vi "Periodic Tasks.vi"(8 "error in":errorcluster) -> ()   [LabVIEW 2017]
doc: "This VI runs in parallel to other robot code. It can contain as many user-defined periodic loops as you need. These can carry out PID or other sorts of timed response."
uses:
  d7755982-491b-4a48-a7ae-66e749655537.vi
  <vilib>/Rock Robotics/WPI/Utilities/WPI_GetSetVariantRefNum.vi
  <vilib>/Rock Robotics/Network Tables/NT Write Boolean.vi
  <vilib>/Rock Robotics/Network Tables/NT Write Number.vi
  <vilib>/Rock Robotics/Network Tables/NT Write Numeric Array.vi
  <vilib>/Rock Robotics/Network Tables/NT Write Boolean Array.vi
  <vilib>/Rock Robotics/SystemInterfaces/AI/FPGA_AIChannel.ctl
  <vilib>/Rock Robotics/WPI/SerialPort/WPI_SerialPort.ctl
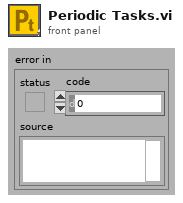
[diagram p1: front panel]
types:
  T1 = typedef "WPI_SerialPort.ctl" = enum16{"Onboard RS-232", "MXP TTL", "USB 1", "USB 2"}
  T2 = typedef "WPI_SerialPortRef.ctl" = cluster{"DevStatus":errorcluster, "Serial Port Name":refnum<visa-resource-name>}
  T3 = typedef "FPGA_AIChannel.ctl" = enum8{"AI 0", "AI 1", "AI 2", "AI 3", "AI MXP 0", "AI MXP 1", "AI MXP 2", "AI MXP 3", "Invalid"}
  T4 = typedef "WPI_AnalogChannelDevRef.ctl" = cluster{"DevStatus":errorcluster, "Analog Channel":T3}
  T5 = typedef "WPI_JoystickDevRef.ctl" = cluster{"Device":T6}
  T6 = typedef "WPI_JoystickDeviceEnum.ctl" = enum16{"USB 0", "USB 1", "USB 2", "USB 3", "USB 4", "USB 5"}
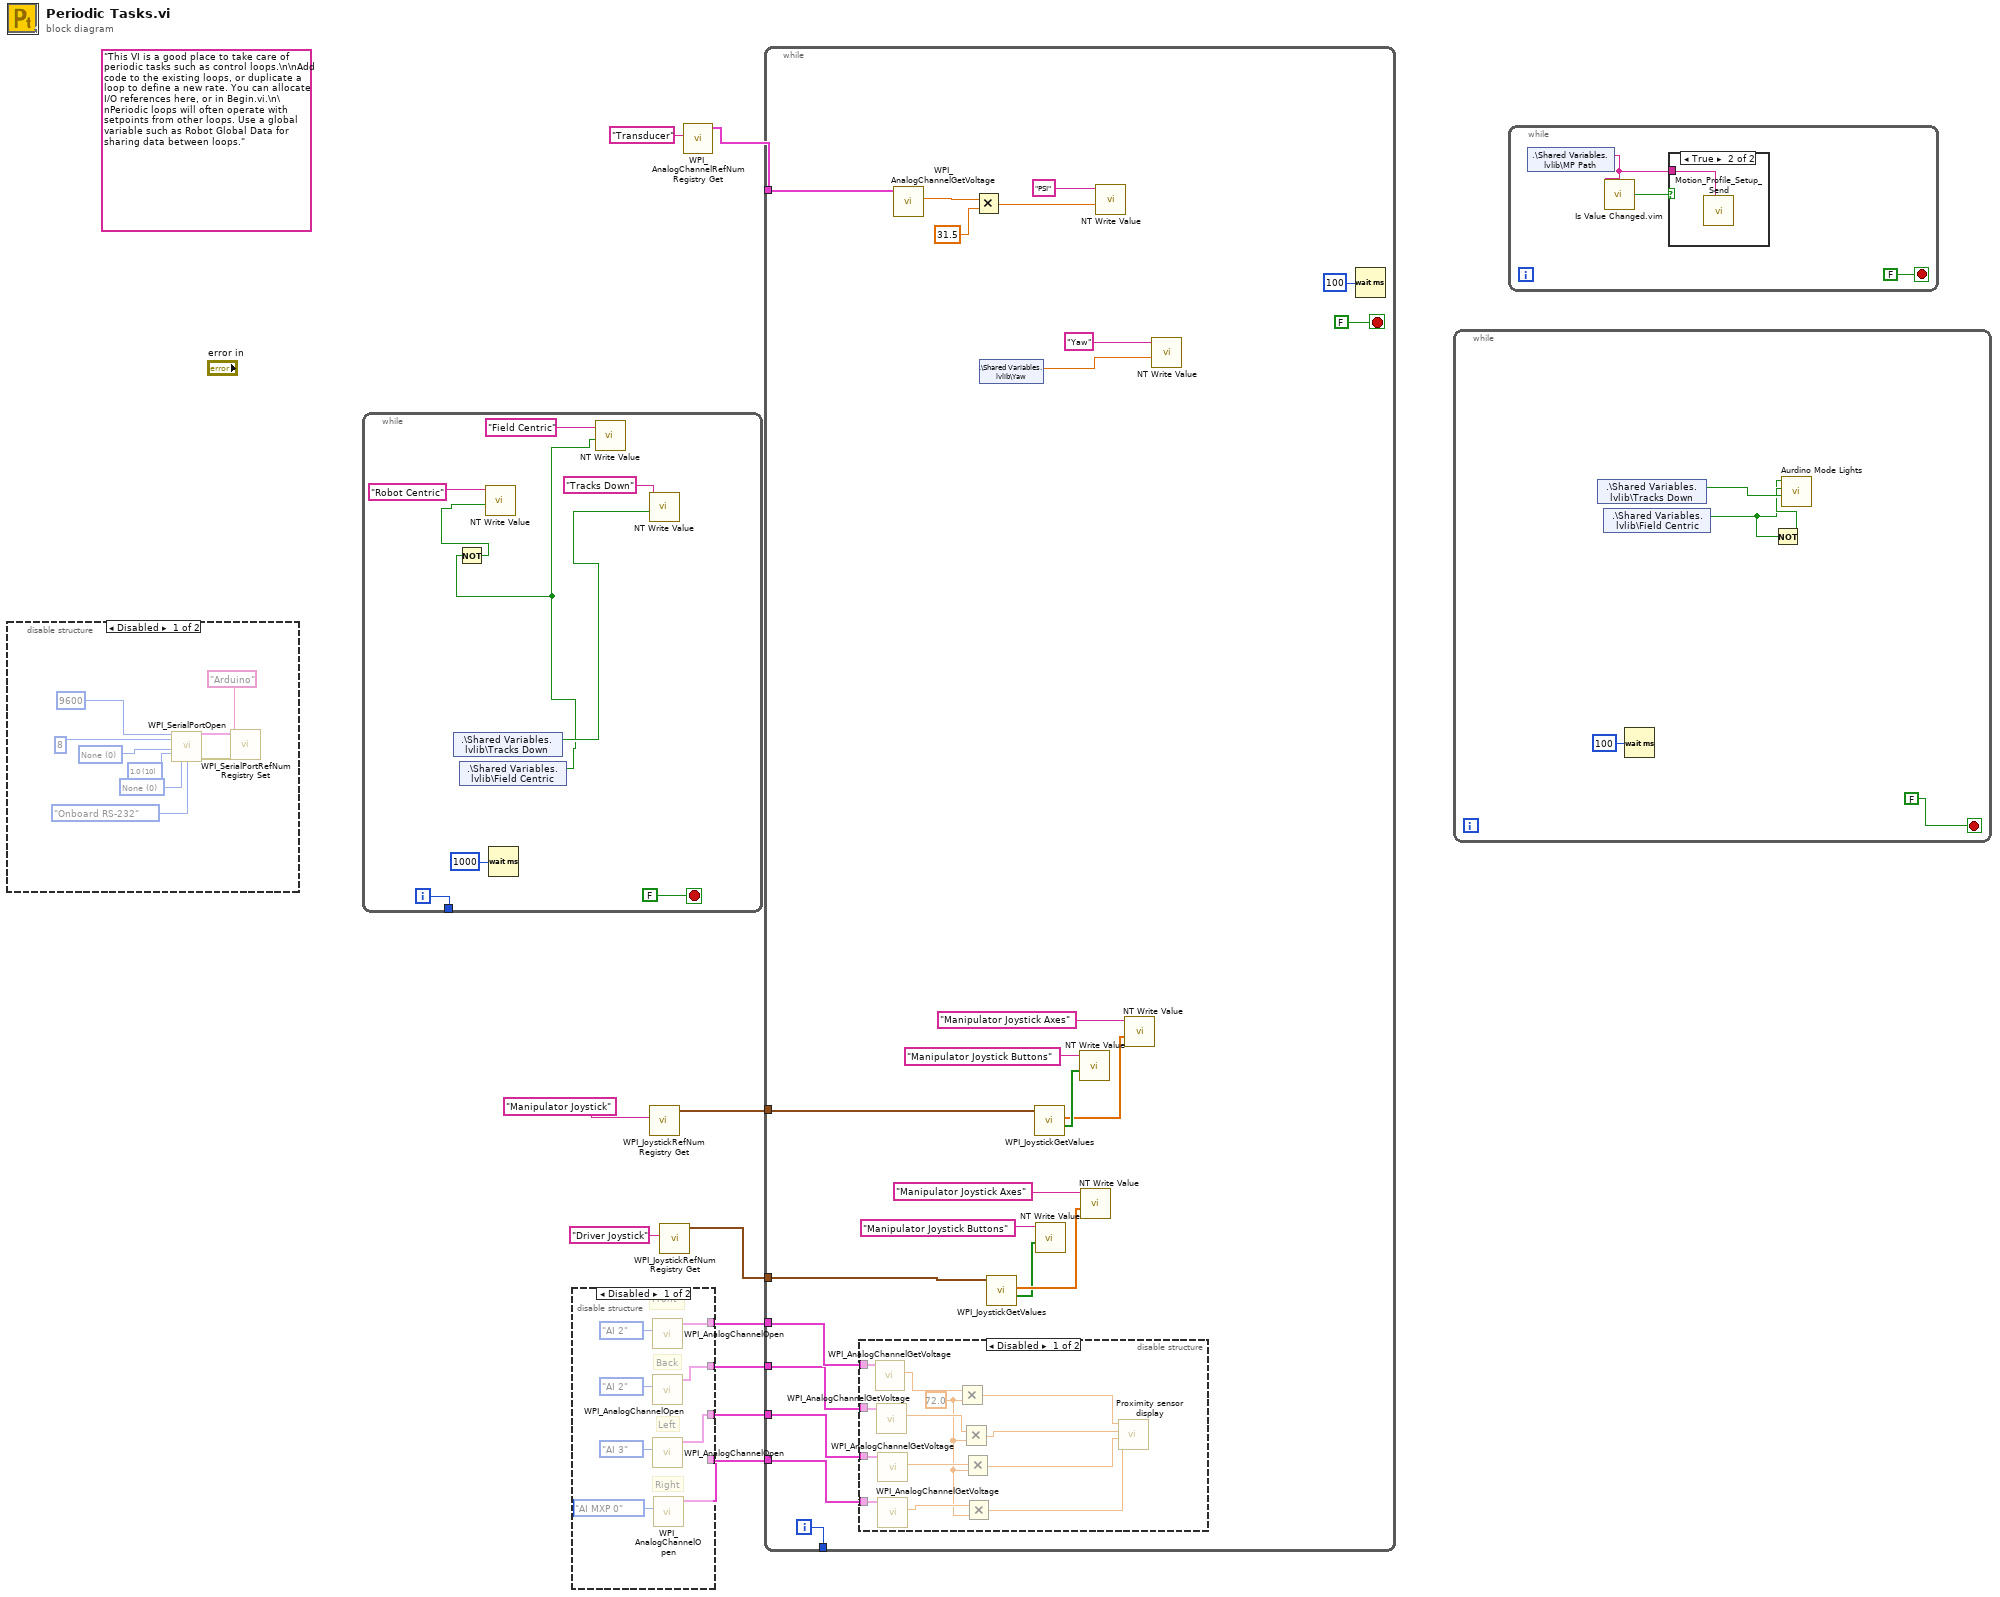
[diagram p0: block diagram]
diagram:
  (unwired) "This VI is a good place to take care of periodic tasks such as control loops.\n\nAdd code to the existing loops, or duplicate a loop to define a new rate. You can allocate I/O references here, or in Begin.vi.\n\nPeriodic loops will often operate with setpoints from other loops. Use a global variable such as Robot Global Data for sharing data between loops."
  n1 = disable-structure shown="Disabled" {
    frame Disabled {
      w12 = u16 0 items=["None", "XON/XOFF", "RTS/CTS", "XON/XOFF & RTS/CTS", "DTR/DSR", "XON/XOFF & DTR/DSR"] ("Flow Control")
      w13 = u16 10 items=["1.0"=10, "1.5"=15, "2.0"=20] ("Stop Bits")
      w14 = u16 0 items=["None", "Odd", "Even", "Mark", "Space"] ("Parity")
      n2 = call <vilib>:"WPI_SerialPortOpen.vi"("Baud Rate"=u32 9600, "Data Bits"=u16 8, "Parity"=w14, "Stop Bits"=w13, "Flow Control"=w12, "Serial Port"=WPI_SerialPort."Onboard RS-232") -> ("SerialPortRef"=w16:T2, "error out"=w11:errorcluster)  [unwired: 8 in]
      n3 = call <vilib>:"WPI_SerialPortRefNum Registry Set.vi"("error in (no error)"=w11, "refnum name"="Arduino", "SerialPortRef"=w16) -> ()  [unwired: 7 in, 2 out]
    }
    frame Enabled {
    }
  }
  n4 = while {
    tunnel: [w27] -> _
    i -> [w27]
    stop <- FALSE stop-if-true
    n5 = shared-variable ".\\Shared Variables.lvlib\\Tracks Down"() -> (w21:bool)  [unwired: 1 in, 1 out]
    n6 = shared-variable ".\\Shared Variables.lvlib\\Field Centric"() -> (w20:bool)  [unwired: 1 in, 1 out]
    n7 = Not(x=w20) -> (.not. x?=w22:bool)
    n8 = call-poly <vilib>:"NT Write Value.vi"("Boolean"=w22, "Name"="Robot Centric") -> ()  [unwired: 9 in, 1 out]
    n9 = Wait (ms)(milliseconds to wait=u32 1000) -> ()  [unwired: 1 out]
    n10 = call-poly <vilib>:"NT Write Value.vi"("Boolean"=w20, "Name"="Field Centric") -> ()  [unwired: 9 in, 1 out]
    n11 = call-poly <vilib>:"NT Write Value.vi"("Boolean"=w21, "Name"="Tracks Down") -> ()  [unwired: 9 in, 1 out]
  }
  n12 = disable-structure shown="Disabled" {
    disable-tunnel: [w33 _] -> w5
    disable-tunnel: [w32 _] -> w4
    disable-tunnel: [w31 _] -> w3
    disable-tunnel: [w30 _] -> w2
    frame Disabled {
      # "Right"
      # "Left"
      # "Back"
      # "Front"
      n13 = call <vilib>:"WPI_AnalogChannelOpen.vi"("Analog Channel"=FPGA_AIChannel."AI 2") -> ("AIDeviceRef"=w33:T4)  [unwired: 9 in, 1 out]
      n14 = call <vilib>:"WPI_AnalogChannelOpen.vi"("Analog Channel"=FPGA_AIChannel."AI 2") -> ("AIDeviceRef"=w32:T4)  [unwired: 9 in, 1 out]
      n15 = call <vilib>:"WPI_AnalogChannelOpen.vi"("Analog Channel"=FPGA_AIChannel."AI 3") -> ("AIDeviceRef"=w31:T4)  [unwired: 9 in, 1 out]
      n16 = call <vilib>:"WPI_AnalogChannelOpen.vi"("Analog Channel"=FPGA_AIChannel."AI MXP 0") -> ("AIDeviceRef"=w30:T4)  [unwired: 9 in, 1 out]
    }
    frame Enabled {
    }
  }
  n17 = call <vilib>:"WPI_JoystickRefNum Registry Get.vi"("refnum name"="Manipulator Joystick") -> ("JoystickDevRef"=w8:T5)  [unwired: 1 in, 9 out]
  n18 = call <vilib>:"WPI_JoystickRefNum Registry Get.vi"("refnum name"="Driver Joystick") -> ("JoystickDevRef"=w6:T5)  [unwired: 1 in, 9 out]
  n19 = call <vilib>:"WPI_AnalogChannelRefNum Registry Get.vi"("refnum name"="Transducer") -> ("AIDeviceRef"=w10:T4)  [unwired: 9 in, 1 out]
  n20 = while {
    tunnel: w10 -> [w58]
    tunnel: [w57] -> _
    tunnel: w8 -> [w51]
    tunnel: w6 -> [w49]
    tunnel: w5 -> [w44]
    tunnel: w4 -> [w43]
    tunnel: w3 -> [w42]
    tunnel: w2 -> [w41]
    i -> [w57]
    stop <- FALSE stop-if-true
    n21 = disable-structure shown="Disabled" {
      disable-tunnel: w44 -> [w64 _]
      disable-tunnel: w43 -> [w63 _]
      disable-tunnel: w42 -> [w62 _]
      disable-tunnel: w41 -> [w61 _]
      frame Disabled {
        w69 = 72.0 ("y")
        n22 = call <vilib>:"WPI_AnalogChannelGetVoltage.vi"("AIDeviceRef"=w64) -> ("Voltage"=w73:dbl)  [unwired: 8 in, 2 out]
        n23 = call <vilib>:"WPI_AnalogChannelGetVoltage.vi"("AIDeviceRef"=w63) -> ("Voltage"=w70:dbl)  [unwired: 8 in, 2 out]
        n24 = call <vilib>:"WPI_AnalogChannelGetVoltage.vi"("AIDeviceRef"=w62) -> ("Voltage"=w72:dbl)  [unwired: 8 in, 2 out]
        n25 = call <vilib>:"WPI_AnalogChannelGetVoltage.vi"("AIDeviceRef"=w61) -> ("Voltage"=w71:dbl)  [unwired: 8 in, 2 out]
        n26 = Multiply(x=w73, y=w69) -> (x*y=w68:dbl)
        n27 = Multiply(x=w70, y=w69) -> (x*y=w67:dbl)
        n28 = Multiply(x=w72, y=w69) -> (x*y=w66:dbl)
        n29 = Multiply(x=w71, y=w69) -> (x*y=w65:dbl)
        n30 = call "Proximity sensor display.vi"("Right Ultrasonic Value"=w65, "Left Ultrasonic Value"=w66, "Back Ultrasonic Value"=w67, "Front Ultrasonic Value"=w68) -> ()  [unwired: 8 in]
      }
      frame Enabled {
      }
    }
    n31 = call <vilib>:"WPI_AnalogChannelGetVoltage.vi"("AIDeviceRef"=w58) -> ("Voltage"=w40:dbl)  [unwired: 8 in, 2 out]
    n32 = Multiply(x=w40, y=31.5) -> (x*y=w39:dbl)
    n33 = shared-variable ".\\Shared Variables.lvlib\\Yaw"() -> (w55:dbl)  [unwired: 1 in, 1 out]
    n34 = call <vilib>:"WPI_JoystickGetValues.vi"("JoystickDevRef"=w49) -> ("Buttons"=w45:bool[], "Axes"=w46:dbl[])  [unwired: 6 in, 3 out]
    n35 = call <vilib>:"WPI_JoystickGetValues.vi"("JoystickDevRef"=w51) -> ("Buttons"=w54:bool[], "Axes"=w50:dbl[])  [unwired: 6 in, 3 out]
    n36 = call-poly <vilib>:"NT Write Value.vi"("Boolean Array"=w45, "Name"="Manipulator Joystick Buttons") -> ()  [unwired: 9 in, 1 out]
    n37 = call-poly <vilib>:"NT Write Value.vi"("Boolean Array"=w54, "Name"="Manipulator Joystick Buttons") -> ()  [unwired: 9 in, 1 out]
    n38 = call-poly <vilib>:"NT Write Value.vi"("Numeric Array"=w46, "Name"="Manipulator Joystick Axes") -> ()  [unwired: 9 in, 1 out]
    n39 = call-poly <vilib>:"NT Write Value.vi"("Numeric"=w39, "Name"="PSI") -> ()  [unwired: 9 in, 1 out]
    n40 = call-poly <vilib>:"NT Write Value.vi"("Numeric Array"=w50, "Name"="Manipulator Joystick Axes") -> ()  [unwired: 9 in, 1 out]
    n41 = call-poly <vilib>:"NT Write Value.vi"("Numeric"=w55, "Name"="Yaw") -> ()  [unwired: 9 in, 1 out]
    n42 = Wait (ms)(milliseconds to wait=u32 100) -> ()  [unwired: 1 out]
  }
  n43 = while {
    stop <- FALSE stop-if-true
    n44 = shared-variable ".\\Shared Variables.lvlib\\Tracks Down"() -> (w78:bool)  [unwired: 1 in, 1 out]
    n45 = shared-variable ".\\Shared Variables.lvlib\\Field Centric"() -> (w76:bool)  [unwired: 1 in, 1 out]
    n46 = Wait (ms)(milliseconds to wait=u32 100) -> ()  [unwired: 1 out]
    n47 = Not(x=w76) -> (.not. x?=w77:bool)
    n48 = call "Aurdino Mode Lights.vi"("Tracks Down"=w78, "Robot Centric"=w77, "Field Centric"=w76) -> ()  [unwired: 7 in]
  }
  n49 = while {
    stop <- FALSE stop-if-true
    n50 = shared-variable ".\\Shared Variables.lvlib\\MP Path"() -> (w79:string)  [unwired: 1 in, 1 out]
    n51 = call "Is Value Changed.vim"("value"=w79) -> ("changed or first call?"=w80:bool)
    n52 = case shown="True" w80 {
      tunnel: w79 -> [_ w82]
      frame False {
      }
      frame True {
        n53 = call "Motion_Profile_Setup_Send.vi"("name or relative path"=w82) -> ()  [unwired: 11 in]
      }
    }
  }
